vi "streamWrite.vi"(8 "error in (no error)":errorcluster, 9 "Front of stream":bool, 10 "String":string, 11 "TextTestRunner in":refnum<class "TextTestRunner.JUnitXML.lvclass">) -> (0 "error out":errorcluster, 3 "TextTestRunner out":refnum<class "TextTestRunner.JUnitXML.lvclass">)   [LabVIEW 2013, in "TextTestRunner.JUnitXML.lvclass"]
uses:
  TextTestRunner.JUnitXML.lvclass
  <vilib>/addons/_JKI Toolkits/VI Tester/TextTestRunner.llb/TextTestRunner.lvclass
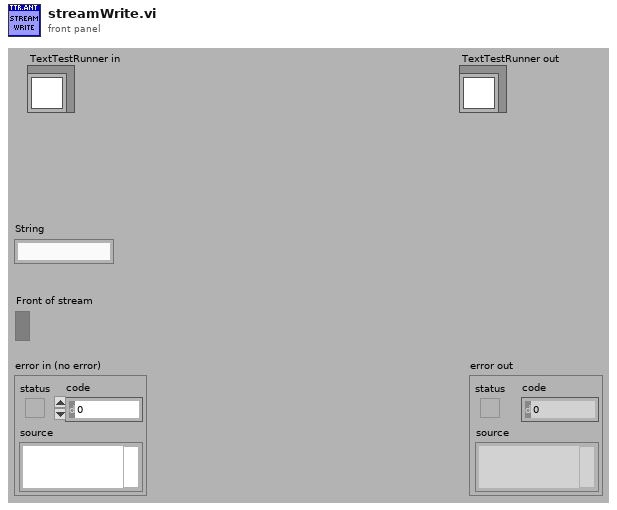
[diagram p1: front panel]
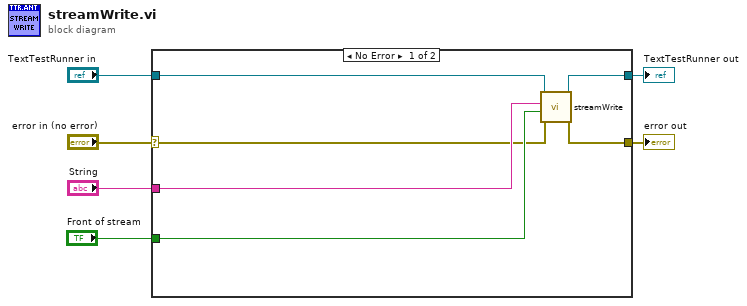
[diagram p0: block diagram]
diagram:
  n1 = case shown="No Error" "error in (no error)" {
    selector: "error in (no error)" -> [w7 w14]
    tunnel: [w8 w14] -> w5
    tunnel: [w11 w13] -> w3
    tunnel: "TextTestRunner in" -> [w12 w13]
    tunnel: "String" -> [w10 _]
    tunnel: "Front of stream" -> [w9 _]
    frame No Error {
      n2 = call-parent "streamWrite.vi"("error in (no error)"=w7, "Front of stream"=w9, "String"=w10, "TextTestRunner in"=w12) -> ("error out"=w8:errorcluster, "TextTestRunner out"=w11:refnum<class "TextTestRunner.JUnitXML.lvclass">)  [unwired: 6 in]
    }
    frame Error {
    }
  }
  "error out" <- w5
  "TextTestRunner out" <- w3
